vi "PCO_GetCameraSetup.vi"(8 "error in (no error)":errorcluster {"code" format="%x"}, 11 "ph":u64) -> (0 "error out":errorcluster {"code" format="%x"}, 2 "ErrorMessage":i32 format="%x", 3 "ph out":u64, 4 "dwSetup":u32[](array[numeric]), 5 "wType":u16)   [LabVIEW 2020, in "SDK.lvlib" / "GeneralCameraControl.lvlib"]
doc: "<b>Description:</b>\nCommand can be used to get the shutter mode of a pco.edge.This function is used to query the current operation mode of the camera. Some cameras can work at different operation modes with different descriptor settings.\n\n<b>Supported camera type:</b>\npco.edge\n\n<b>Descriptor dependency:</b>\nNone"
uses:
  GeneralCameraControl.lvlib
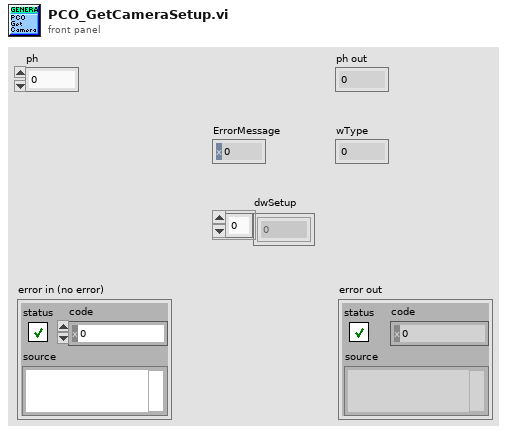
[diagram p1: front panel]
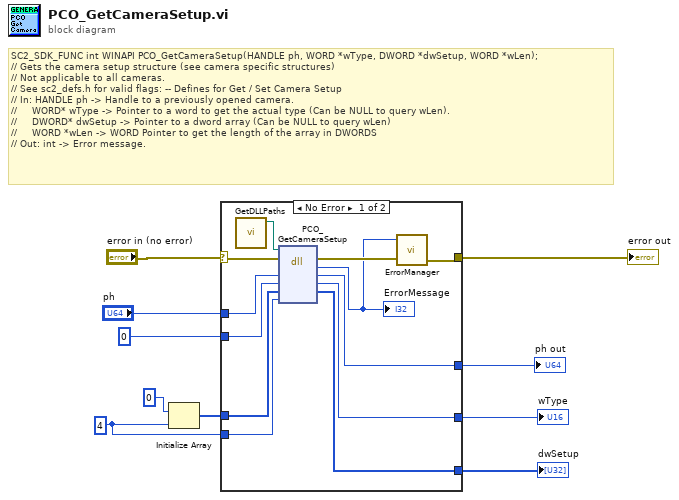
[diagram p0: block diagram]
diagram:
  w1 = u16 4
  # "SC2_SDK_FUNC int WINAPI PCO_GetCameraSetup(HANDLE ph, WORD *wType, DWORD *dwSetup, WORD *wLen);\n// Gets the camera setup structure (see camera specific structures)\n// Not applicable to all cameras.\n// See sc2_defs.h for valid flags: -- Defines for Get / Set Camera Setup\n// In: HANDLE ph -> Handle to a previously opened camera.\n//     WORD* wType -> Pointer to a word to get the actual type (Can be NULL to query wLen).\n//     DWORD* dwSetup -> Pointer to a dword array (Can be NULL to query wLen)\n//     WORD *wLen -> WORD Pointer to get the length of the array in DWORDS\n// Out: int -> Error message."
  n1 = Initialize Array(u32 0 ("element"), w1) -> (w2:u32[])
  n2 = case shown="No Error" "error in (no error)" {
    selector: "error in (no error)" -> [w18 w26]
    tunnel: "ph" -> [w22 w25]
    tunnel: [w21 w25] -> w9
    tunnel: [w19 w26] -> w8
    tunnel: [w16 w23] -> w6
    tunnel: [w15 w24] -> w5
    tunnel: u16 0 ("wType") -> [w14 w24]
    tunnel: w1 -> [w13 _]
    tunnel: w2 -> [w12 w23]
    frame No Error {
      n3 = call "GetDLLPaths.vi"() -> ("SC2_Cam_Path"=w11:path)  [unwired: 9 in, 2 out]
      n4 = dll-call lib="?" fn="PCO_GetCameraSetup"(path in=w11, error in=w18, "ph"=w22, "wType"=w14, "dwSetup"=w12, "wLen"=w13) -> (error out=w20:errorcluster, "return type"=w17:i32, "ph"=w21:u64, "wType"=w15:u16, "dwSetup"=w16:u32[])  [unwired: 2 in, 1 out]
      "ErrorMessage" <- w17
      n5 = call "ErrorManager.vi"("error in (no error)"=w20, "error code"=w17) -> ("error out"=w19:errorcluster)  [unwired: 3 in]
    }
    frame Error {
    }
  }
  "ph out" <- w9
  "error out" <- w8
  "wType" <- w5
  "dwSetup" <- w6
